vi "write2Byte Tx Rx.vi"(6 "data":u16, 7 "address":u16, 8 "error in (no error)":errorcluster, 9 "id":u8, 10 "protocol_version":i32, 11 "port_num":i32) -> (0 "error out":errorcluster)   [LabVIEW 2018, in "labview.lvlib"]
doc: "WINDECLSPEC void write2ByteTxRx (int port_num, int protocol_version, uint8_t id, uint16_t address, uint16_t data);"
uses:
  labview.lvlib
  dxl_x86_c.dll
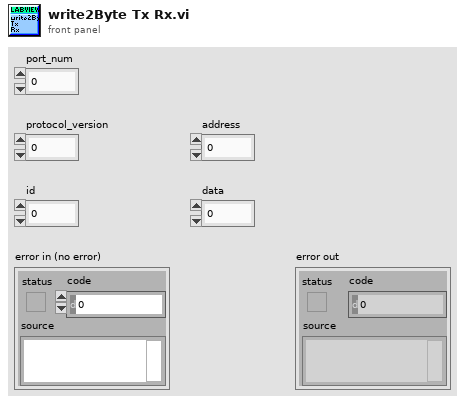
[diagram p1: front panel]
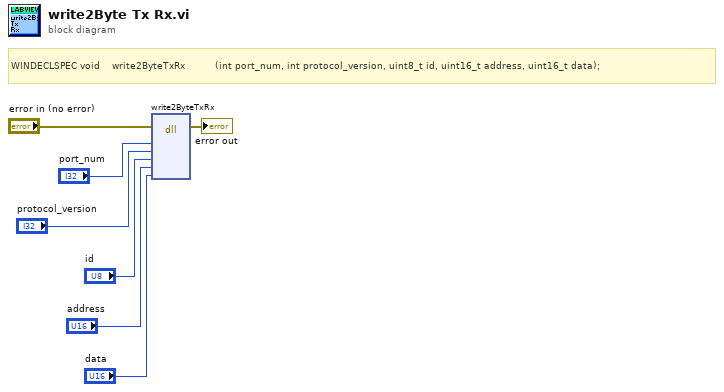
[diagram p0: block diagram]
diagram:
  # "WINDECLSPEC void    write2ByteTxRx          (int port_num, int protocol_version, uint8_t id, uint16_t address, uint16_t data);"
  n1 = dll-call lib="C:/Users/joaos/OneDrive/Documents/[PhD]/Project Omnidirectional Vehicle/Vanes/LabView_code/joaoandthethreestands/DynamixelSDK-3.7.31/labview/new_compilation/dxl_x86_c.*" fn="write2ByteTxRx"(error in="error in (no error)", "port_num"="port_num", "protocol_version"="protocol_version", "id"="id", "address"="address", "data"="data") -> (error out=→"error out":errorcluster)  [unwired: 8 in, 1 out]
